vi "Adquisicion de voltaje y corriente.vi"() -> ()   [LabVIEW 2019]
uses:
  Control 1.ctl
  <vilib>/Waveform/WDTOps.llb/WDT Append Waveforms DBL.vi
panel:
  out "Velocidad medida (rpm)":dbl
  out "Frecuencia":dbl
  in  "Stop":bool=TRUE
  in  "Control de Caragas":T1(ring)
  in  "Motor a analizar":dbl
  out "Torque":dbl
  out "Torque":dbl(knob) scale=-10.0..10.0
  out "Corriente generado":dynamicdata(graph)
  out "Corriente":dbl
  out "Voltaje":dbl
  out "Corriente RMS":dbl(knob) scale=0.0..2.0
  in  "stop (F)":T2 caption="Parar"
  out "Voltaje generado":dynamicdata(graph)
  out "Voltaje RMS":dbl(knob) scale=0.0..230.0
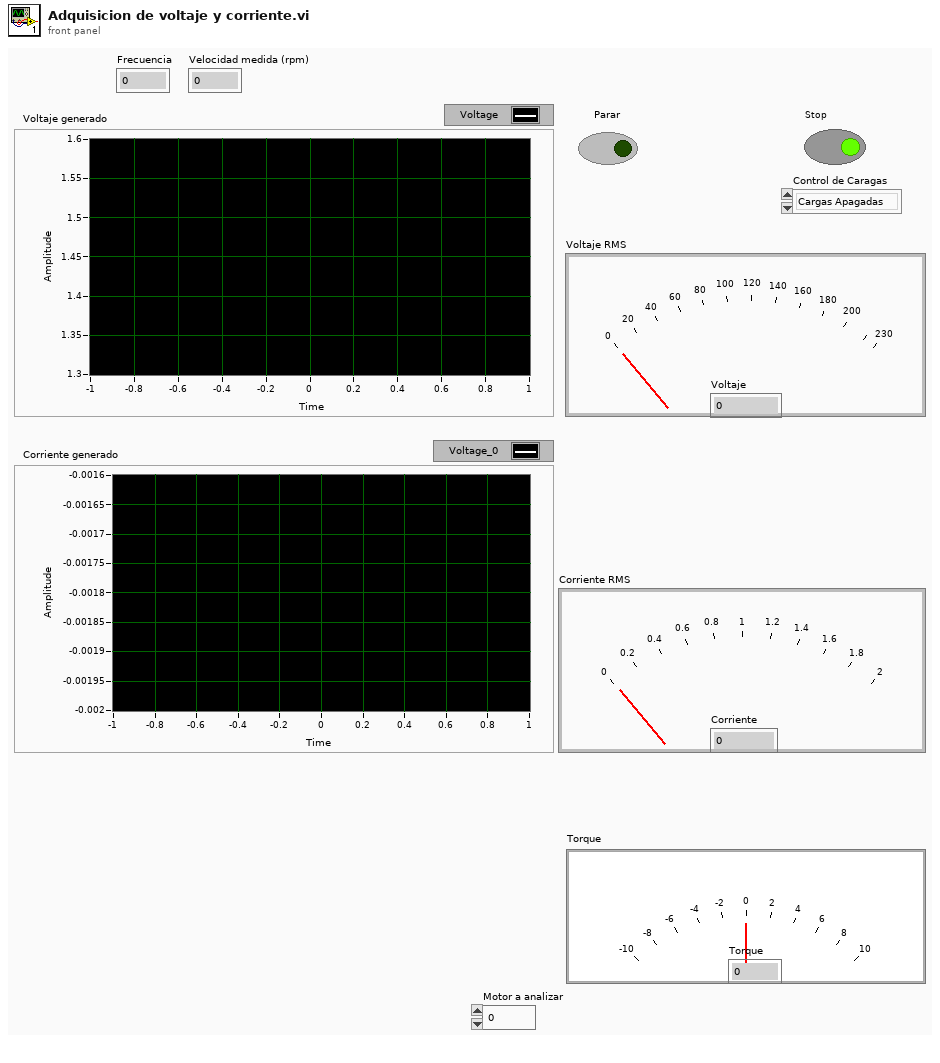
[diagram p1: front panel]
types:
  T1 = enum16{"Cargas Apagadas", "Activar Primer Carga", "Activar Segunda Carga", "Activar Ambas Cargas"}
  T2 = typedef "Control 1.ctl" = bool
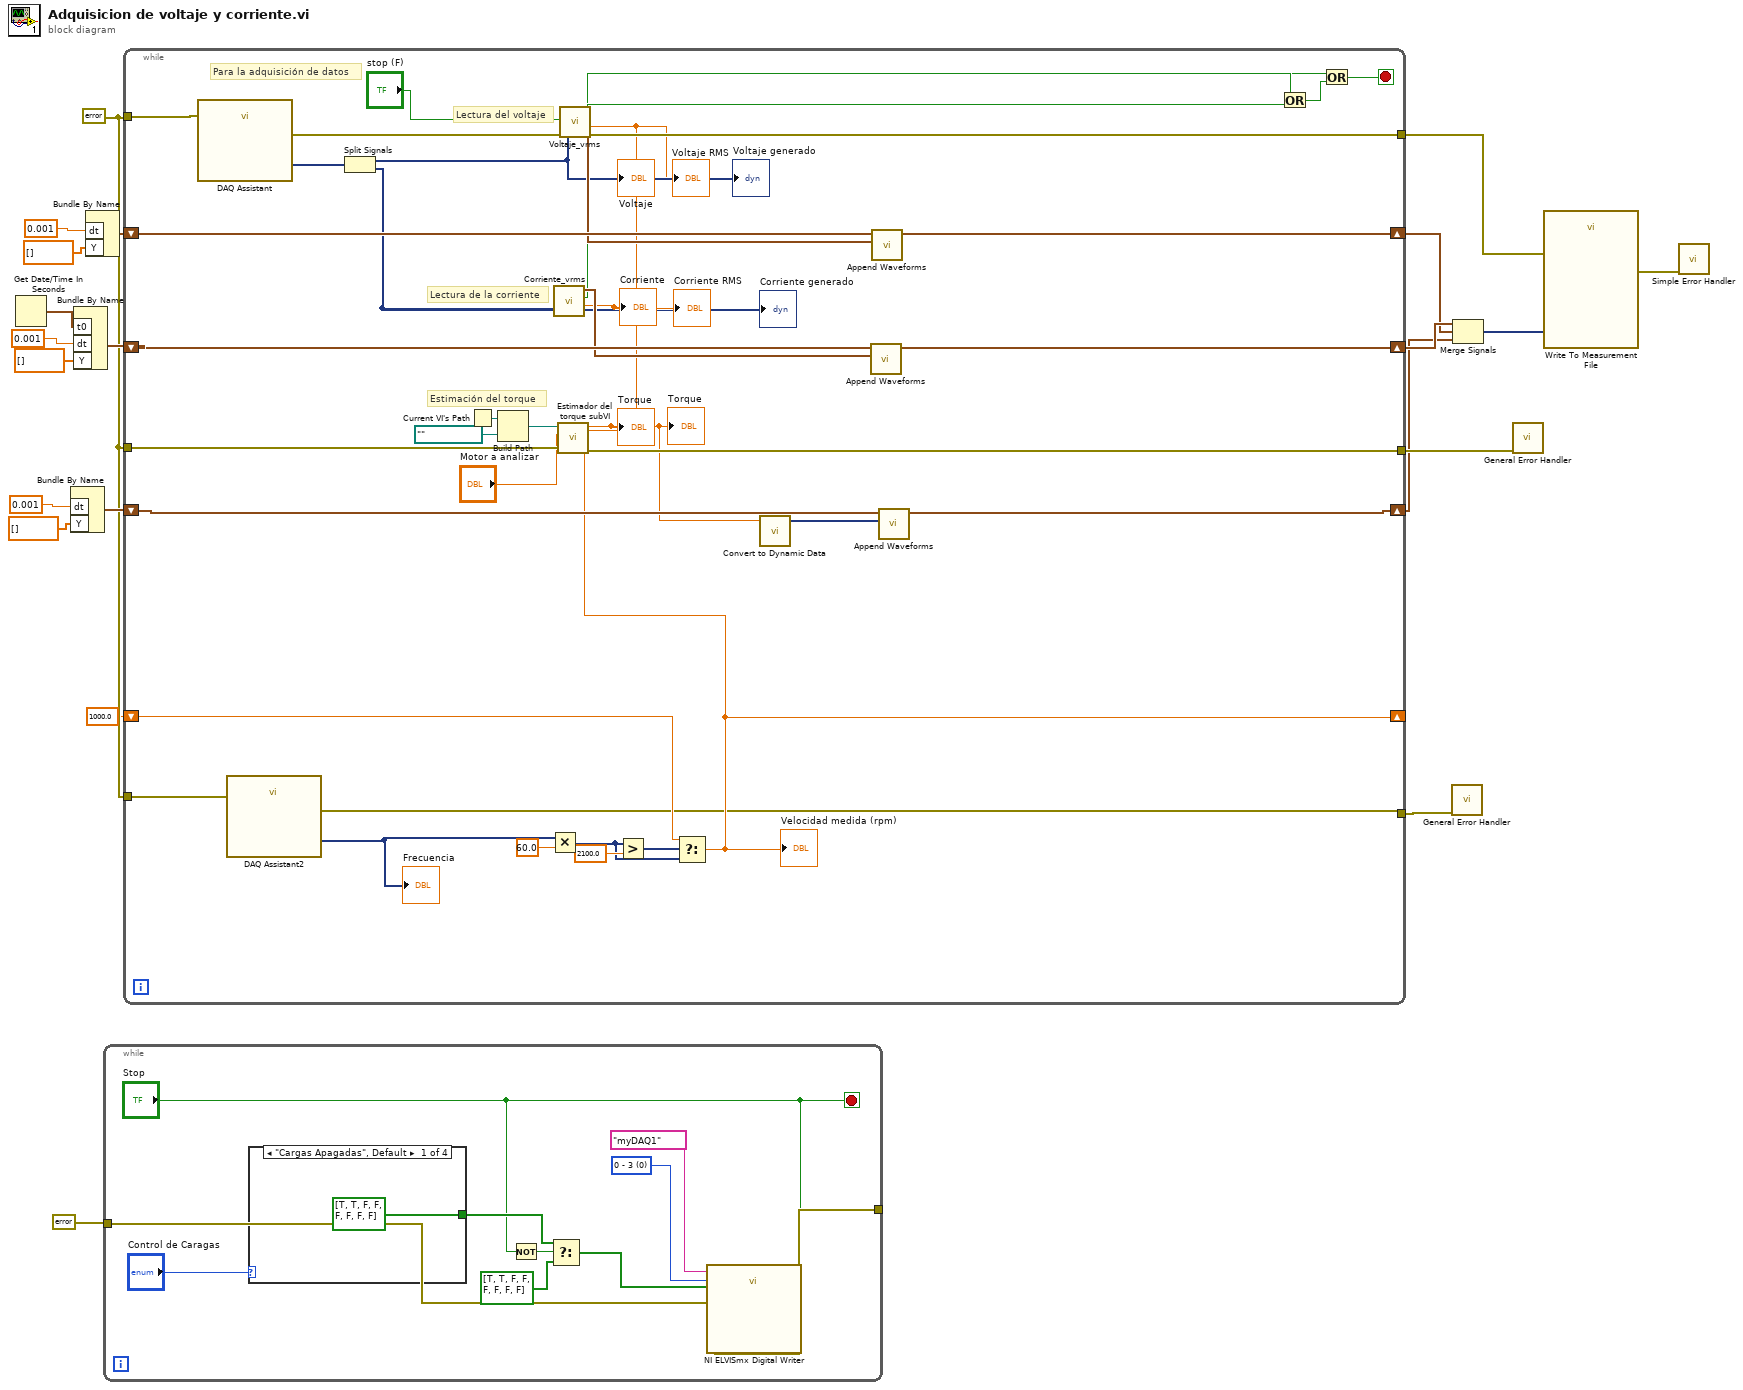
[diagram p0: block diagram]
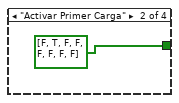
[diagram p2: hidden frame]
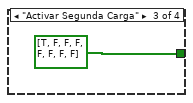
[diagram p3: hidden frame]
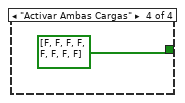
[diagram p4: hidden frame]
diagram:
  w3 = errorcluster {"status"=FALSE, "code"=0, "source"=""} ("error in")
  n1 = Get Date/Time In Seconds() -> (seconds since 1Jan1904=w19:timestamp)
  n2 = Bundle By Name("dt"=0.001, "Y"=dbl[] []) -> (w9:waveform(dbl))  [unwired: 1 in]
  n3 = Bundle By Name("t0"=w19, "dt"=0.001, "Y"=dbl[] []) -> (w18:waveform(dbl))  [unwired: 1 in]
  n4 = Bundle By Name("dt"=0.001, "Y"=dbl[] []) -> (w13:waveform(dbl))  [unwired: 1 in]
  n5 = while {
    tunnel: errorcluster {"status"=FALSE, "code"=0, "source"=""} ("error in") -> [w24]
    tunnel: [w23] -> _
    stop <- "Stop" stop-if-true
    w25 = u16 0 items=["0 - 3", "4 - 7", "0 - 7"] ("myDAQ Lines to Write")
    n6 = case shown="\"Cargas Apagadas\", Default" "Control de Caragas" {
      tunnel: [bool[] [TRUE, TRUE, FALSE, FALSE, FALSE, FALSE, FALSE, FALSE] ("DO Lines") bool[] [FALSE, TRUE, FALSE, FALSE, FALSE, FALSE, FALSE, FALSE] ("DO Lines") bool[] [TRUE, FALSE, FALSE, FALSE, FALSE, FALSE, FALSE, FALSE] ("DO Lines") bool[] [FALSE, FALSE, FALSE, FALSE, FALSE, FALSE, FALSE, FALSE] ("DO Lines")] -> w29
      frame "Cargas Apagadas", Default {
      }
      frame "Activar Primer Carga" {
      }
      frame "Activar Segunda Carga" {
      }
      frame "Activar Ambas Cargas" {
      }
    }
    n7 = Not(x="Stop") -> (.not. x?=w30:bool)
    n8 = Select(t=w29, s=w30, f=bool[] [TRUE, TRUE, FALSE, FALSE, FALSE, FALSE, FALSE, FALSE] ("DO Lines")) -> (s? t:f=w26:bool[])
    n9 = call "NI ELVISmx Digital Writer"("Device Name"=tag "myDAQ1", "myDAQ Lines to Write"=w25, "Stop"="Stop", "DO Lines"=w26, "error in"=w24) -> ("error out"=w23:errorcluster)  [unwired: 14 in]
  }
  n10 = while {
    tunnel: w3 -> [w39]
    shift-right: [w73] -> w17
    shift-left: w18 -> [w70]
    tunnel: [w72] -> w5
    shift-right: [w71] -> w16
    shift-left: w13 -> [w69]
    tunnel: w3 -> [w56]
    tunnel: [w54] -> w12
    shift-right: [w52] -> w8
    shift-left: w9 -> [w51]
    tunnel: w3 -> [w36]
    tunnel: [w38] -> w1
    shift-right: [w42] -> _
    shift-left: 1000.0 -> [w44]
    stop <- w68 stop-if-true
    # "Para la adquisición de datos"
    # "Estimación del torque"
    # "Lectura de la corriente"
    # "Lectura del voltaje"
    n11 = call "DAQ Assistant"("error in"=w39) -> ("data"=w41:dynamicdata, "error out"=w40:errorcluster)  [unwired: 16 in, 1 out]
    n12 = call "DAQ Assistant2"("error in"=w36) -> ("data"=w37:dynamicdata, "error out"=w38:errorcluster)  [unwired: 16 in, 1 out]
    "Frecuencia" <- w37
    n13 = Split Signals(w41) -> (w66:dynamicdata, w60:dynamicdata)  [unwired: 2 in]
    "Voltaje generado" <- w66
    "Corriente generado" <- w60
    n14 = Current VI's Path() -> (path=w59:path)
    n15 = Build Path(base path=w59, name or relative path=path "") -> (appended path=w57:path)
    n16 = Multiply(x=w37, y=60.0) -> (x*y=w45:dynamicdata)
    n17 = call "Corriente_vrms.vi"("Dynamic Data"=w60) -> ("Scalar"=→"Corriente RMS" →"Corriente":dbl, "Boolean"=w63:bool, "Waveform"=w65:waveform(dbl))  [unwired: 8 in]
    n18 = call "Voltaje_vrms.vi"("error in (no error)"=w40, "data"=w66) -> ("error out"=w72:errorcluster, "Scalar"=w55:dbl, "Waveform"=w67:waveform(dbl), "Boolean"=w62:bool)  [unwired: 6 in]
    "Voltaje RMS" <- w55
    "Voltaje" <- w55
    n19 = Greater?(x=w45, y=2100.0) -> (0:w46:dynamicdata)
    n20 = Select(t=w44, s=w46, f=w45) -> (s? t:f=w42:dbl)
    "Velocidad medida (rpm)" <- w42
    n21 = call "Estimador del torque subVI.vi"("Real"=w55, "error in (no error)"=w56, "Real 2"=w42, "Real 3"="Motor a analizar", "appended path"=w57) -> ("error out"=w54:errorcluster, "Numeric"=w49:dbl)  [unwired: 5 in]
    "Torque" <- w49
    "Torque" <- w49
    n22 = call "Convert to Dynamic Data"("Double"=w49) -> ("Dynamic Data Type"=w50:dynamicdata)  [unwired: 3 in]
    n23 = call-poly <vilib>:"Append Waveforms.vi"("waveform B"=w65, "waveform A"=w70) -> ("waveform out"=w73:waveform(dbl))  [unwired: 8 in, 1 out]
    n24 = call-poly <vilib>:"Append Waveforms.vi"("waveform B"=w67, "waveform A"=w69) -> ("waveform out"=w71:waveform(dbl))  [unwired: 8 in, 1 out]
    n25 = call-poly <vilib>:"Append Waveforms.vi"("waveform B"=w50, "waveform A"=w51) -> ("waveform out"=w52:waveform(dbl))  [unwired: 8 in, 1 out]
    n26 = Or(x=w62, y=w63) -> (x .or. y?=w61:bool)
    n27 = Or(x="stop (F)", y=w61) -> (x .or. y?=w68:T2)
  }
  n28 = call <vilib>:"General Error Handler.vi"("error in (no error)"=w1) -> ()  [unwired: 10 in, 5 out]
  n29 = Merge Signals(w17, w16, w8) -> (w7:dynamicdata)
  n30 = call <vilib>:"General Error Handler.vi"("error in (no error)"=w12) -> ()  [unwired: 10 in, 5 out]
  n31 = call "Write To Measurement File"("Signals"=w7, "error in (no error)"=w5) -> ("error out"=w6:errorcluster)  [unwired: 15 in, 2 out]
  n32 = call <vilib>:"Simple Error Handler.vi"("error in (no error)"=w6) -> ()  [unwired: 4 in, 5 out]
